vi "Calculate Optimal Height.vi"(8 "error in (no error)":errorcluster, 9 "Max Height (200)":u32=200, 10 "Target Width (300)":u32=300, 11 "Dialog in":refnum<class "Dialog.lvclass">) -> (0 "error out":errorcluster, 1 "Set Height":u32, 2 "VScrollbar Visible?":bool, 3 "Dialog out":refnum<class "Dialog.lvclass">, 4 "Optimal Height":u32)   [LabVIEW 2012, in "Dialog.lvlib" / "Dialog.lvclass"]
uses:
  Dialog.lvclass
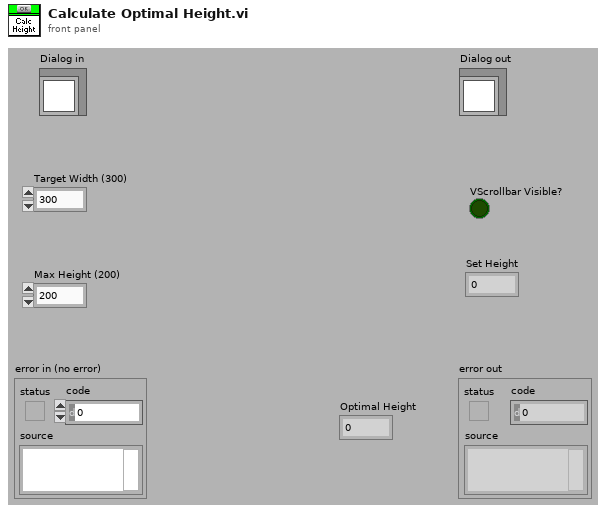
[diagram p1: front panel]
types:
  T1 = typedef "LVBoundsTypeDef.ctl" = cluster{"Width":u32, "Height":u32}
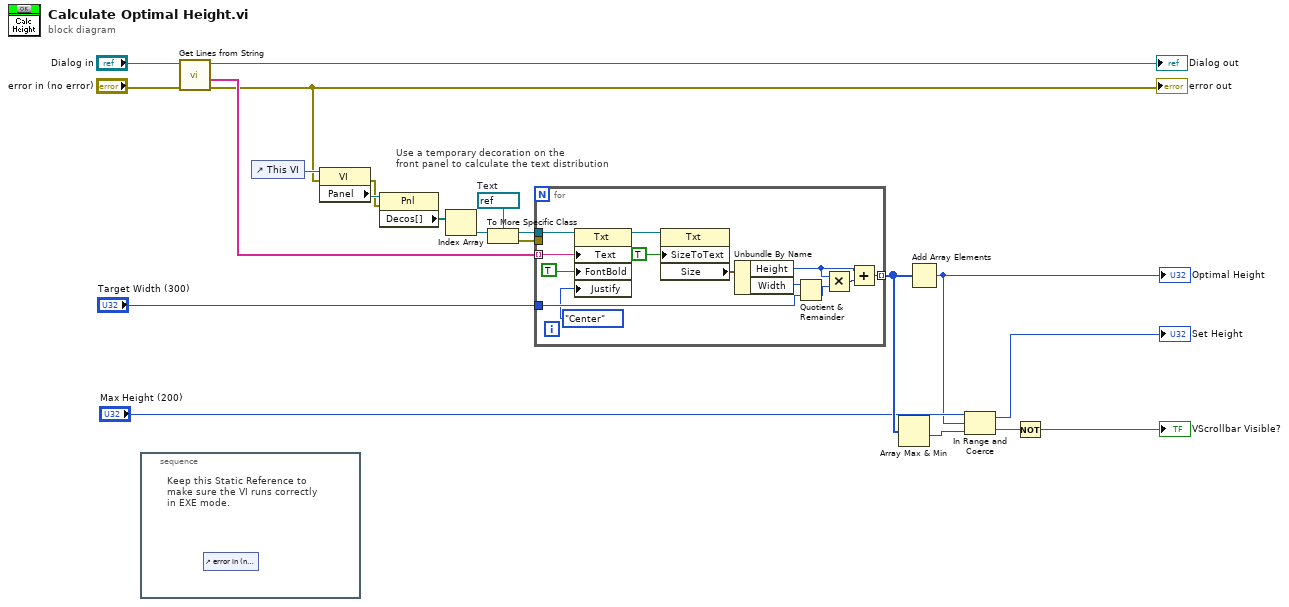
[diagram p0: block diagram]
diagram:
  w21 = refnum<vi> refnum  # Text
  # "Use a temporary decoration on the\nfront panel to calculate the text distribution"
  n1 = stacked-sequence {
    frame #0 {
      # "Keep this Static Reference to\nmake sure the VI runs correctly\nin EXE mode."
      n2 = control-ref of="error in (no error)"() -> ()  [unwired: 1 out]
    }
  }
  n3 = call-dynamic "Get Lines from String.vi"("error in (no error)"="error in (no error)", "Dialog in"="Dialog in") -> ("error out"=w1:errorcluster, "Lines"=w8:string[], "Dialog out"=→"Dialog out":refnum<class "Dialog.lvclass">)  [unwired: 7 out]
  "error out" <- w1
  n4 = control-ref of="This VI"() -> (w17:refnum<vi>)
  n5 = property class="VI"(reference=w17, error in=w1) -> (error out=w3:errorcluster, "Panel"=w18:refnum<vi>)  [unwired: 1 out]
  n6 = property class="Pnl"(reference=w18, error in=w3) -> ("Decos[]"=w19:refnum<vi>[])  [unwired: 2 out]
  n7 = Index Array(array=w19) -> (element=w20:refnum<vi>)  [unwired: 1 in]
  n8 = To More Specific Class(target class=w21, reference=w20) -> (specific class reference=w12:refnum<vi>, error out=w2:errorcluster)  [unwired: 1 in]
  n9 = for {
    tunnel: "Target Width (300)" -> [w33]
    tunnel: [w30] -> w14 mode=indexing
    tunnel: w12 -> [w25]
    tunnel: w8 -> [w24] mode=indexing
    tunnel: w2 -> [_]
    n10 = property class="Txt"(reference=w25, "Text"=w24, "FontBold"=TRUE ("Font:Bold"), "Justify"=enum16{"Left", "Center", "Right"}."Center" ("Justification")) -> (reference out=w29:refnum<vi>)  [unwired: 1 in, 1 out]
    n11 = property class="Txt"(reference=w29, "SizeToText"=TRUE ("Size to Text?")) -> ("Size"=w26:T1)  [unwired: 1 in, 2 out]
    n12 = Unbundle By Name(w26) -> ("Height"=w22:u32, "Width"=w34:u32)
    n13 = Quotient & Remainder(x=w34, y=w33) -> (floor(x/y)=w32:u32)  [unwired: 1 out]
    n14 = Multiply(x=w22, y=w32) -> (x*y=w31:u32)
    n15 = Add(x=w22, y=w31) -> (x+y=w30:u32)
  }
  n16 = Array Max & Min(array=w14) -> (min value=w15:u32)  [unwired: 3 out]
  n17 = Add Array Elements(numeric array=w14) -> (sum=w6:u32)
  "Optimal Height" <- w6
  n18 = In Range and Coerce(upper limit="Max Height (200)", x=w6, lower limit=w15) -> (coerced(x)=→"Set Height":u32, In Range?=w16:bool)
  n19 = Not(x=w16) -> (.not. x?=→"VScrollbar Visible?":bool)
